vi "Validate Addressable Endpoints.vi"(8 "error in (no error)":errorcluster, 11 "Hardware Ref in":T1 format="%.0x") -> (0 "error out":errorcluster, 3 "Hardware Ref out":T1 format="%.0x")   [LabVIEW 2019, in "Routing and Faulting Hardware API.lvlib"]
doc: "Asserts that the list of addressable endpoints has been set for the given Hardware Custom Device."
uses:
  Routing and Faulting Hardware API.lvlib
  <vilib>/NI VeriStand/Custom Device API/Custom Device Item Ref.ctl
  Routing and Faulting Hardware API Constants.vi
  <vilib>/NI VeriStand/Custom Device API/Custom Device API.lvlib
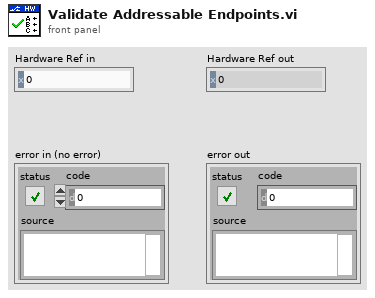
[diagram p1: front panel]
types:
  T1 = typedef "Custom Device API.lvlib/Custom Device Item Ref.ctl" = u64
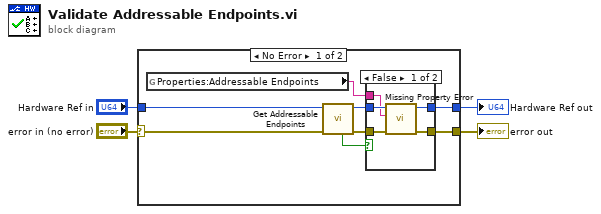
[diagram p0: block diagram]
diagram:
  n1 = case shown="No Error" "error in (no error)" {
    selector: "error in (no error)" -> [w7 w21]
    tunnel: [w11 w20] -> w4
    tunnel: [w9 w21] -> w3
    tunnel: "Hardware Ref in" -> [w6 w20]
    frame No Error {
      n2 = global read "Routing and Faulting Hardware API Constants.vi" "Properties:Addressable Endpoints"() -> (w12:string)
      n3 = call "Get Addressable Endpoints.vi"("error in (no error)"=w7, "Hardware Ref in"=w6) -> ("error out"=w8:errorcluster, "Hardware Ref out"=w10:T1, "Found?"=w5:bool)  [unwired: 6 in, 1 out]
      n4 = case shown="False" w5 {
        tunnel: w8 -> [w17 w19]
        tunnel: [w16 w19] -> w9
        tunnel: w10 -> [w15 w18]
        tunnel: [w14 w18] -> w11
        tunnel: w12 -> [w13 _]
        frame False {
          n5 = call "Missing Property Error.vi"("error in (no error)"=w17, "Property Name"=w13, "Hardware Ref in"=w15) -> ("error out"=w16:errorcluster, "Hardware Ref out"=w14:T1)  [unwired: 7 in]
        }
        frame True {
        }
      }
    }
    frame Error {
    }
  }
  "Hardware Ref out" <- w4
  "error out" <- w3
